vi "Curvature.vi"() -> ()   [LabVIEW 2018]
panel:
  out "X":dbl
  in  "Robot Y":dbl
  in  "Robot X":dbl
  in  "Robot Heading":dbl
  in  "Look Ahead Y":dbl
  in  "Look Ahead X":dbl
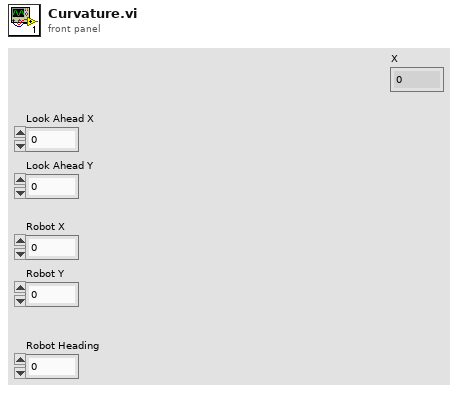
[diagram p1: front panel]
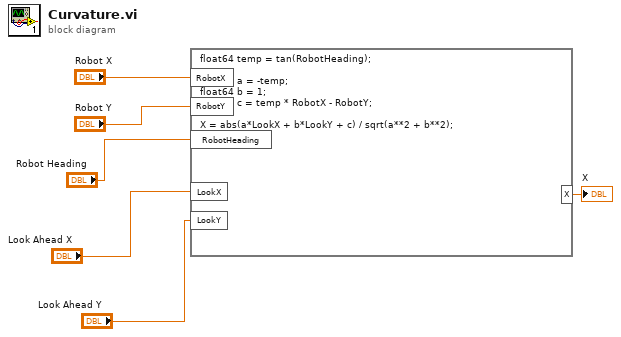
[diagram p0: block diagram]
diagram:
  n1 = formula code="float64 temp = tan(RobotHeading);\n\nfloat64 a = -temp;\nfloat64 b = 1;\nfloat64 c = temp * RobotX - RobotY;\n\nX = abs(a*LookX + b*LookY + c) / sqrt(a**2 + b**2);"("RobotX"="Robot X", "RobotY"="Robot Y", "LookX"="Look Ahead X", "LookY"="Look Ahead Y", "RobotHeading"="Robot Heading") -> ("X"=→"X":dbl)
